vi "Delete Active DUT Connector Band.vi"(7 "RX (RX0)":i32(ring) items=["RX0", "RX1", "RX2", "RX3", "None"], 8 "error in (no error)":errorcluster, 9 "TX (TX0)":i32(ring) items=["TX0", "TX1", "None"], 10 "ConnectorName (\"Connector1\")":string="Connector1", 11 "VISA resource name":refnum<visa-resource-name>) -> (0 "error out":errorcluster, 3 "VISA resource name out":refnum<visa-resource-name>)   [LabVIEW 2020, in "Rohde&Schwarz CMXP Base.lvlib"]
doc: "Removes frequency bands from an antenna connector of the active DUT (connector-centric approach).\n\nYou can remove several bands with a single command. Specify the technology and the band number for each band.\n\nAttribute:\n-\n\nRemote-control command:\nREMove:DUT:CONNector:BAND"
uses:
  <instrlib>/Rohde&Schwarz CMXP Base/Rohde&Schwarz CMXP Base.lvlib
  <instrlib>/Rohde&Schwarz CMXP Base/Private/rsidr_core.llb/rsidr_core.lvlib
panel:
  in  "Bands":cluster{"Type (LTE)":i32, "Band Number":i32}[](array[cluster]) {"Type (LTE)" items=["LTE", "New Radio", "WLAN"]}
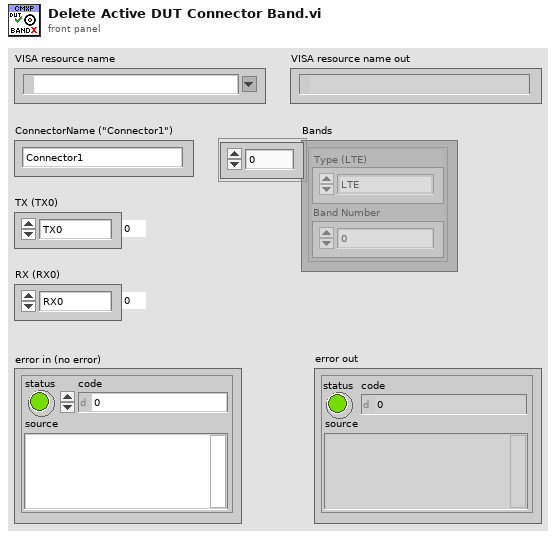
[diagram p1: front panel]
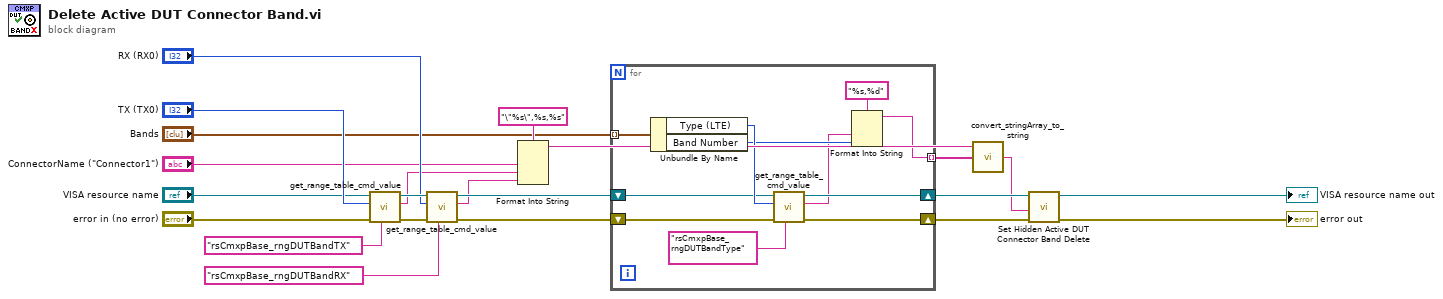
[diagram p0: block diagram]
diagram:
  n1 = call <instrlib>:"get_range_table_cmd_value.vi"("Range Table ID in"="rsCmxpBase_rngDUTBandTX", "error in"="error in (no error)", "Input Int32 value"="TX (TX0)", "VISA resource name"="VISA resource name") -> ("error out"=w22:errorcluster, "Cmd value out"=w6:string, "VISA resource name out"=w21:refnum<visa-resource-name>)  [unwired: 5 in]
  n2 = call <instrlib>:"get_range_table_cmd_value.vi"("Range Table ID in"="rsCmxpBase_rngDUTBandRX", "error in"=w22, "Input Int32 value"="RX (RX0)", "VISA resource name"=w21) -> ("error out"=w4:errorcluster, "Cmd value out"=w5:string, "VISA resource name out"=w19:refnum<visa-resource-name>)  [unwired: 5 in]
  n3 = Format Into String(format string="\"%s\",%s,%s", "ConnectorName (\"Connector1\")", w6, w5) -> (resulting string=w3:string)  [unwired: 2 in, 1 out]
  n4 = for {
    tunnel: "Bands" -> [w33] mode=indexing
    tunnel: [w23] -> w2 mode=indexing
    shift-right: [w26] -> w17
    shift-left: w19 -> [w30]
    shift-right: [w25] -> w18
    shift-left: w4 -> [w32]
    n5 = Unbundle By Name(w33) -> ("Type (LTE)"=w31:i32, "Band Number"=w27:i32)
    n6 = call <instrlib>:"get_range_table_cmd_value.vi"("Range Table ID in"="rsCmxpBase_rngDUTBandType", "error in"=w32, "Input Int32 value"=w31, "VISA resource name"=w30) -> ("error out"=w25:errorcluster, "Cmd value out"=w24:string, "VISA resource name out"=w26:refnum<visa-resource-name>)  [unwired: 5 in]
    n7 = Format Into String(format string="%s,%d", w24, w27) -> (resulting string=w23:string)  [unwired: 2 in, 1 out]
  }
  n8 = call <instrlib>:"convert_stringArray_to_string.vi"("string array in"=w2, "String to add before (\"\")"=w3) -> ("string out"=w1:string)  [unwired: 3 in]
  n9 = call "Set Hidden Active DUT Connector Band Delete"("error in (no error)"=w18, "Hidden Active DUT Connector Band Delete ()"=w1, "instrument handle"=w17) -> ("error out"=→"error out":errorcluster, "instrument handle out"=→"VISA resource name out":refnum<visa-resource-name>)  [unwired: 7 in]
